vi "TestRUSHShoot.vi"() -> ()   [LabVIEW 2012]
panel:
  in  "ShootConstFlipper":cluster{"Down":dbl, "Up":dbl}={"Down"=0.2, "Up"=0.8}
  in  "ShootFlipperPE":bool
  in  "In Cluster":T1
  out "Out Cluster":T2
  in  "ShootRollerSpd":dbl(slide) scale=-1.0..1.0
  in  "Ground":bool
  in  "Set 4":bool
  in  "ShootConstElev":T3={"1"=2.0, "2"=3.0, "3"=3.5, "4"=4.0, "Ground"=1.0}
  in  "Set 3":bool
  in  "Set 2":bool
  in  "Set 1":bool
  in  "ShootTargetInfo":T4
  in  "Deadband":dbl=0.1
  in  "Default Wheel Speed":dbl=0.75
  in  "IndexerSpeed":dbl=0.5
  in  "ShootManualElev":dbl(slide) scale=-1.0..1.0
  in  "ShootPOTElev":dbl(slide) scale=0.0..5.0
  in  "ShootIndexerEnable":bool
  in  "ShootStartWheels":bool
  in  "ShootTrackEnable":bool
  # "Roller Speed IN"
  # "Roller OUT"
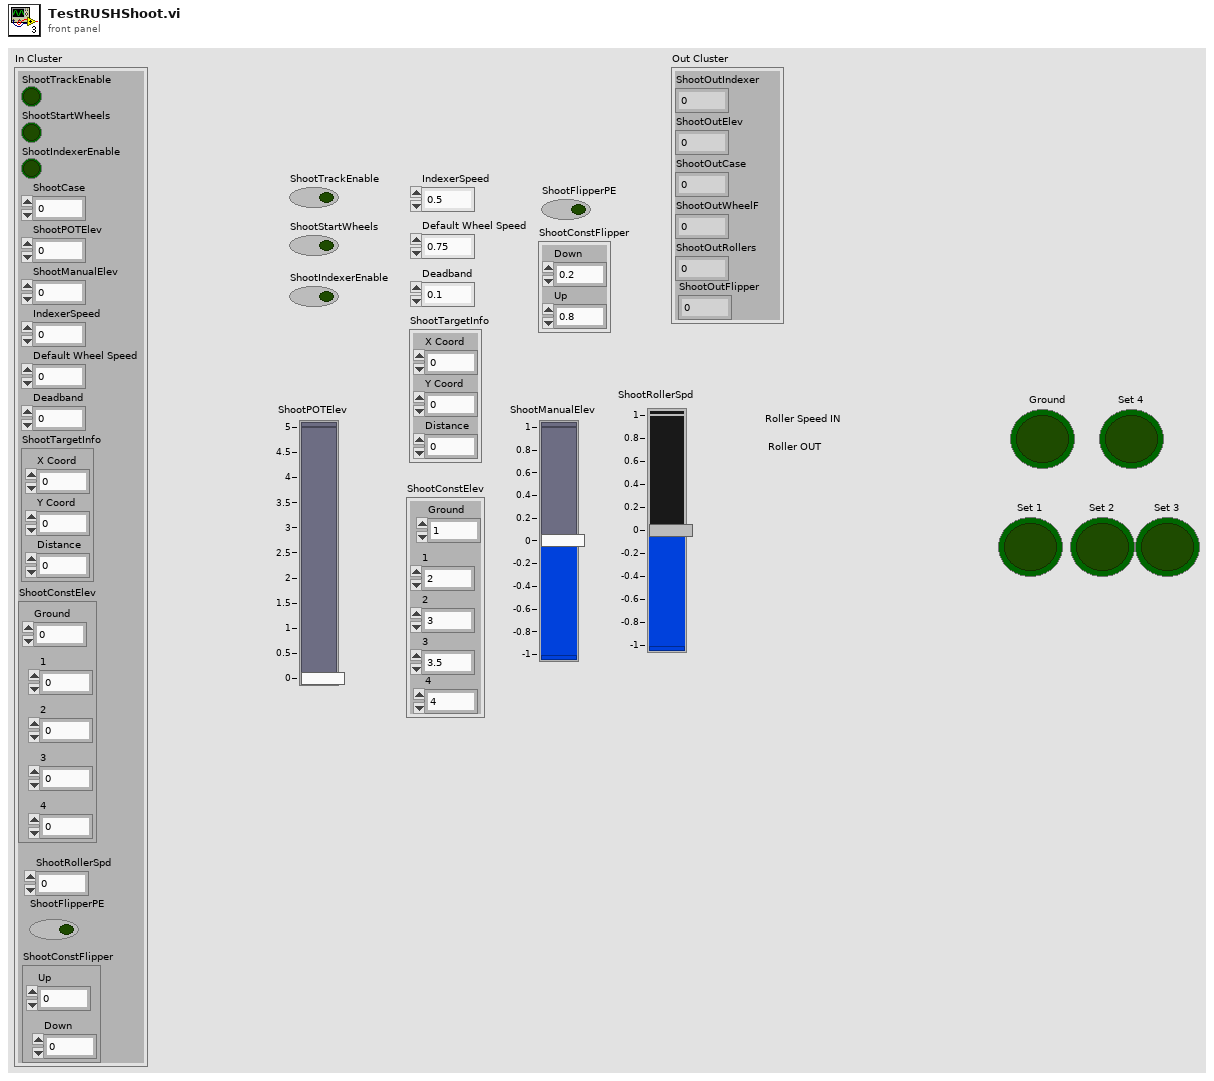
[diagram p1: front panel]
types:
  T1 = cluster{"ShootTrackEnable":bool, "ShootStartWheels":bool, "ShootIndexerEnable":bool, "ShootCase":dbl, "ShootPOTElev":dbl, "ShootManualElev":dbl, "IndexerSpeed":dbl, "Default Wheel Speed":dbl, "Deadband":dbl, "ShootTargetInfo":cluster{"X Coord":dbl, "Y Coord":dbl, "Distance":dbl}, "ShootConstElev":cluster{"1":dbl, "2":dbl, "3":dbl, "4":dbl, "Ground":dbl}, "ShootRollerSpd":dbl, "ShootFlipperPE":bool, "ShootConstFlipper":cluster{"Down":dbl, "Up":dbl}}
  T2 = cluster{"ShootOutIndexer":dbl, "ShootOutElev":dbl, "ShootOutCase":dbl, "ShootOutWheelF":dbl, "ShootOutRollers":dbl, "ShootOutFlipper":dbl}
  T3 = cluster{"1":dbl, "2":dbl, "3":dbl, "4":dbl, "Ground":dbl}
  T4 = cluster{"X Coord":dbl, "Y Coord":dbl, "Distance":dbl}
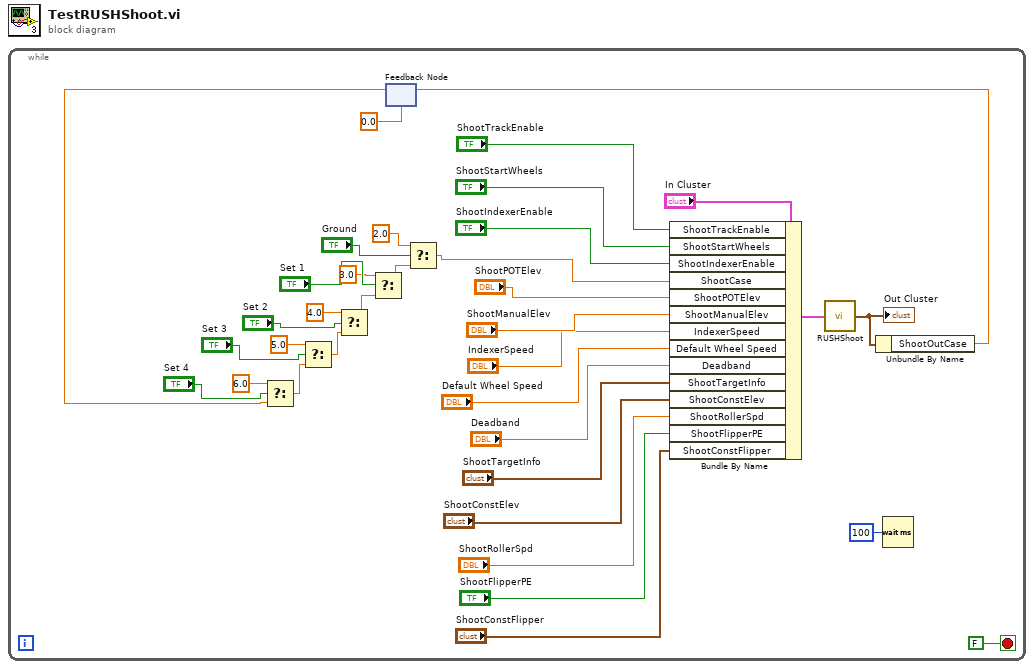
[diagram p0: block diagram]
diagram:
  n1 = while {
    stop <- FALSE stop-if-true
    n2 = feedback #1(0.0 ("ShootOutCase")) -> (w7:dbl)
    n3 = Select(t=6.0, s="Set 4", f=w7) -> (s? t:f=w13:dbl)
    n4 = Select(t=5.0, s="Set 3", f=w13) -> (s? t:f=w32:dbl)
    n5 = Select(t=4.0, s="Set 2", f=w32) -> (s? t:f=w31:dbl)
    n6 = Select(t=3.0, s="Set 1", f=w31) -> (s? t:f=w9:dbl)
    n7 = Select(t=2.0, s="Ground", f=w9) -> (s? t:f=w12:dbl)
    n8 = Bundle By Name(cluster="In Cluster", "ShootTrackEnable"="ShootTrackEnable", "ShootStartWheels"="ShootStartWheels", "ShootIndexerEnable"="ShootIndexerEnable", "ShootCase"=w12, "ShootPOTElev"="ShootPOTElev", "ShootManualElev"="ShootManualElev", "IndexerSpeed"="IndexerSpeed", "Default Wheel Speed"="Default Wheel Speed", "Deadband"="Deadband", "ShootTargetInfo"="ShootTargetInfo", "ShootConstElev"="ShootConstElev", "ShootRollerSpd"="ShootRollerSpd", "ShootFlipperPE"="ShootFlipperPE", "ShootConstFlipper"="ShootConstFlipper") -> (w3:T1)
    n9 = call "RUSHShoot.vi"("In Cluster"=w3) -> ("Out Cluster"=w18:T2)
    "Out Cluster" <- w18
    n10 = Unbundle By Name(w18) -> ("ShootOutCase"=w8:dbl)
    n11 = feedback-in #1(w8) -> ()
    n12 = Wait (ms)(milliseconds to wait=u32 100) -> ()  [unwired: 1 out]
  }
